vi "SaveDataOfDCSignal.vi"() -> ()   [LabVIEW 2019]
panel:
  in  "Write To Text File":bool
  out "Current Iteration":i32
  in  "Stop the Process":bool
  out "Peak to Peak":dbl
  out "Waveform Graph":dynamicdata(graph)
  out "Warning Light":bool
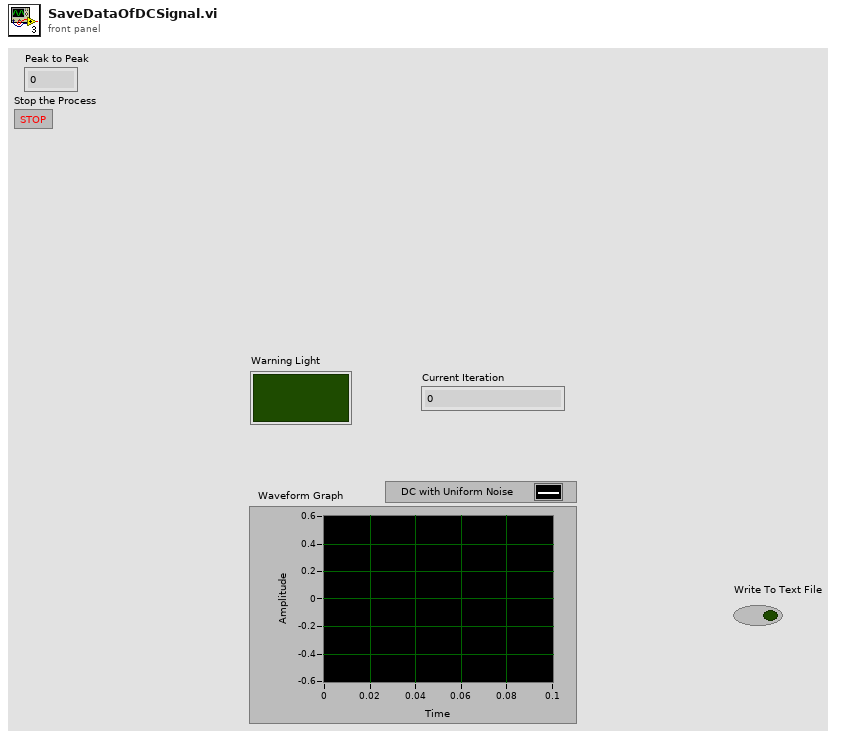
[diagram p1: front panel]
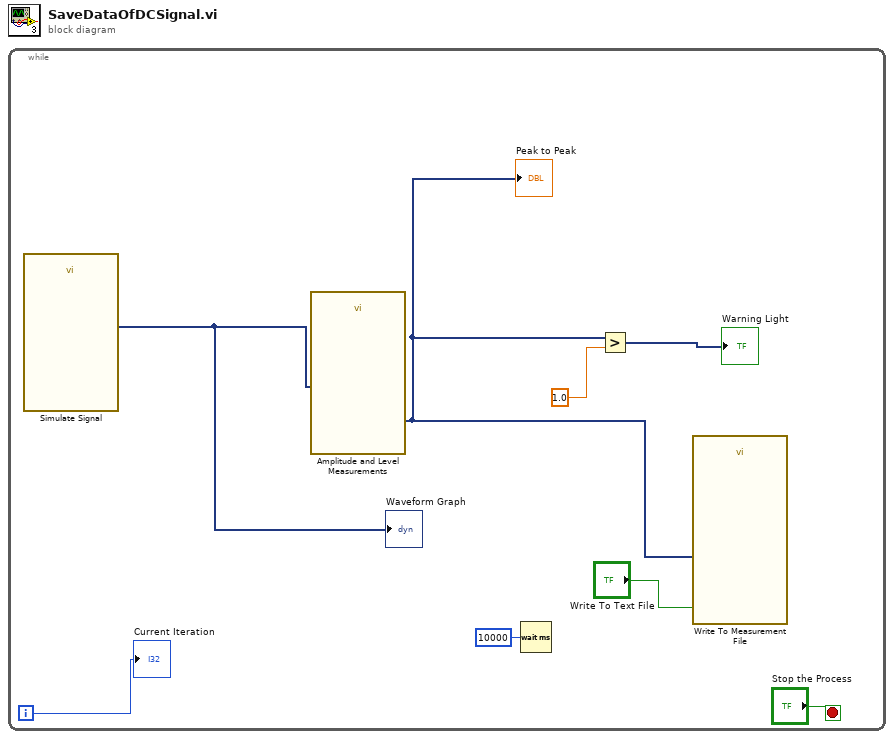
[diagram p0: block diagram]
diagram:
  n1 = while {
    i -> [w4]
    stop <- "Stop the Process" stop-if-true
    n2 = call "Simulate Signal"() -> ("DC with Uniform Noise"=w8:dynamicdata)  [unwired: 14 in, 1 out]
    "Waveform Graph" <- w8
    n3 = call "Amplitude and Level Measurements"("Signals"=w8) -> ("Peak to Peak"=w1:dynamicdata)  [unwired: 13 in, 1 out]
    "Peak to Peak" <- w1
    n4 = Wait (ms)(milliseconds to wait=u32 10000) -> ()  [unwired: 1 out]
    n5 = Greater?(x=w1, y=1.0) -> (0:→"Warning Light":dynamicdata)
    n6 = call "Write To Measurement File"("Signals"=w1, "Enable"="Write To Text File") -> ()  [unwired: 15 in, 3 out]
    "Current Iteration" <- w4
  }
